vi "export method.vi"   [LabVIEW 2012]
uses:
  logic buffer cmd.ctl
types:
  T1 = typedef "logic buffer cmd.ctl" = enum16{"read", "write ouput settings", "write rules", "write setpoints", "write output descriptions", "write all", "calculate setpoints", "save", "open", "Load all setpoint code", "Load one setpoint code", "Configure one setpoint code"}
  T2 = typedef "variable setpoint.ctl" = cluster{"name":string, "unit":string, "value":dbl, "Type":enum16{"Constant", "Variable"}, "variable":cluster{"selected sensors":i32[], "selected set points":i32[], "VI":path, "Data average interval":T3, "code ref":T4}}
  T3 = typedef "data ave interval.ctl" = dbl
  T4 = typedef "type specifier for control code.ctl" = refnum<vi>
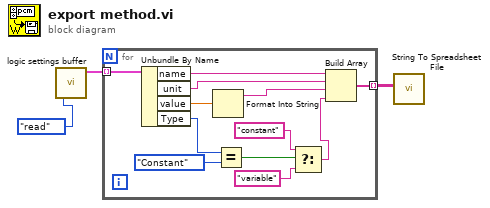
[diagram p0: block diagram]
diagram:
  n1 = call "logic settings buffer.vi"("command"=logic_buffer_cmd."read") -> ("Set Points out"=w2:T2[])  [unwired: 11 in, 7 out]
  n2 = for {
    tunnel: w2 -> [w15] mode=indexing
    tunnel: [w4] -> w1 mode=indexing
    n3 = Unbundle By Name(w15) -> ("name"=w13:string, "unit"=w12:string, "value"=w14:dbl, "Type"=w10:enum16{"Constant", "Variable"})
    n4 = Format Into String(w14) -> (resulting string=w11:string)  [unwired: 3 in, 1 out]
    n5 = Equal?(x=w10, y=enum16{"Constant", "Variable"}."Constant") -> (x = y?=w8:bool)
    n6 = Select(t="constant", s=w8, f="variable") -> (s? t:f=w5:string)
    n7 = Build Array(w13, w12, w11, w5) -> (w4:string[])
  }
  n8 = call "String To Spreadsheet File.vi"("2D data"=w1) -> ()  [unwired: 7 in, 1 out]
